vi "reshape array (Ballard-1553-messages).vi"(10 "index requested":i32=2, 11 "messages in":map{string, T1}[](array[numeric])) -> (3 "messages out":map{string, T1}[](array[numeric]))   [LabVIEW 2020]
uses:
  1553/_controls/aim1553_messages.ctl
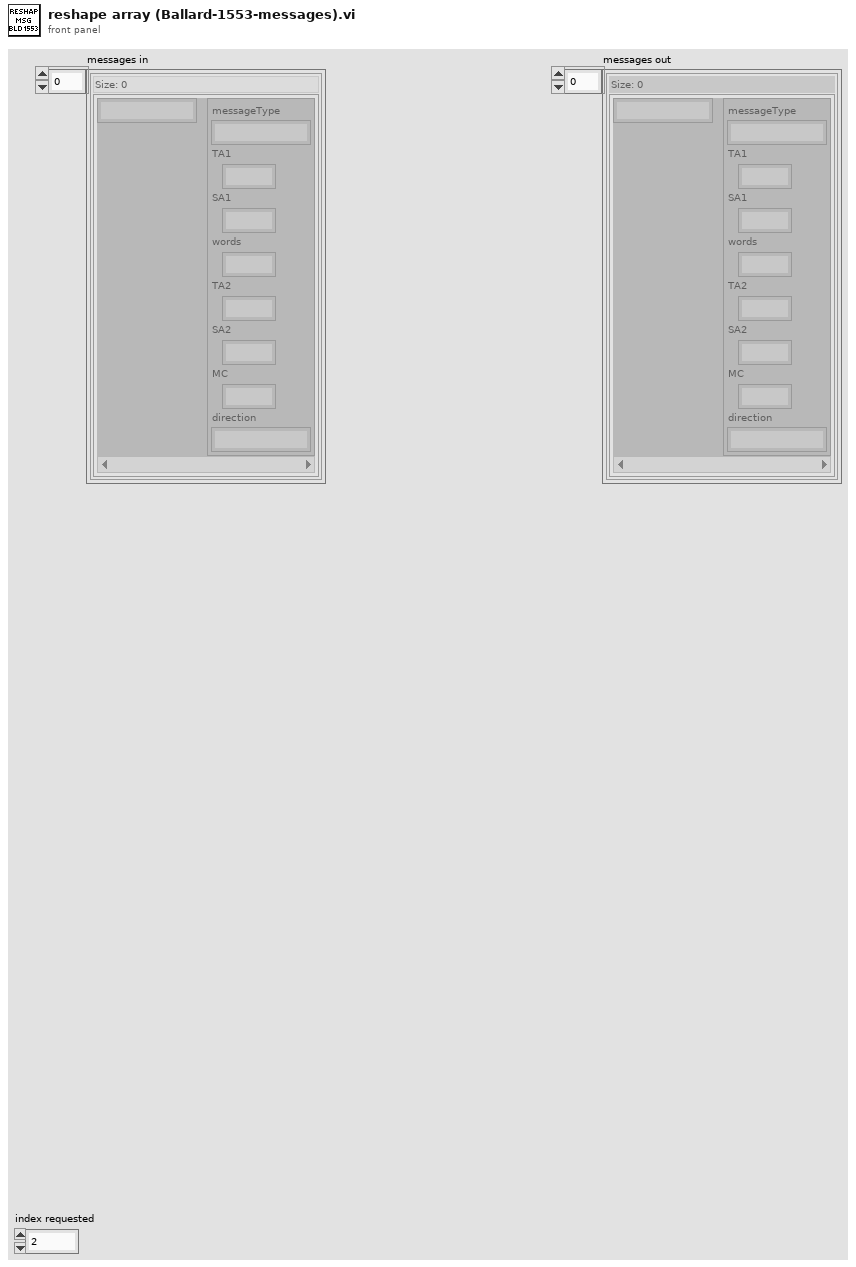
[diagram p1: front panel]
types:
  T1 = typedef "aim1553_messages.ctl" = cluster{"messageType":string, "TA1":i32, "SA1":i32, "words":i32, "TA2":i32, "SA2":i32, "MC":i32, "direction":string}
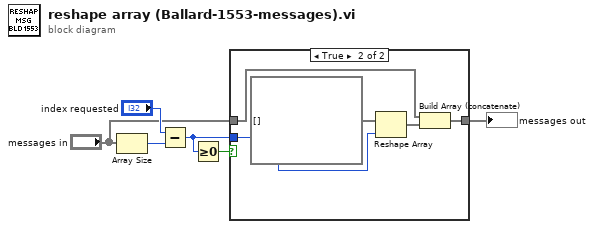
[diagram p0: block diagram]
diagram:
  n1 = Array Size(array="messages in") -> (size(s)=w5:i32)
  n2 = Subtract(x="index requested", y=w5) -> (x-y=w3:i32)
  n3 = Greater Or Equal To 0?(x=w3) -> (x >= 0?=w4:bool)
  n4 = case shown="True" w4 {
    tunnel: w3 -> [_ w12]
    tunnel: "messages in" -> [w7 w10]
    tunnel: [w7 w9] -> w1
    frame False {
    }
    frame True {
      n5 = Reshape Array(map{string, T1}[] [] ("messages in 2"), w12) -> (w11:map{string, T1}[])
      n6 = Build Array (concatenate)(w10, w11) -> (w9:map{string, T1}[])
    }
  }
  "messages out" <- w1
